vi "PH_Cont-601k_PSU.Set Device Readyness.vi"(0 "VI in":refnum<vi>, 2 "Readyness Device to set":T1, 5 "error in (no error)":errorcluster) -> (14 "VI out":refnum<vi>, 19 "error out":errorcluster)   [LabVIEW 2014, in "PH_Cont-601k_PSU.lvlib"]
doc: "This VI sets the Device readyness to own oattributes and indicates it at the GUI."
uses:
  PH_Cont-601k_PSU.lvlib
  PH_Cont-601k_PSU.Readyness Device.ctl
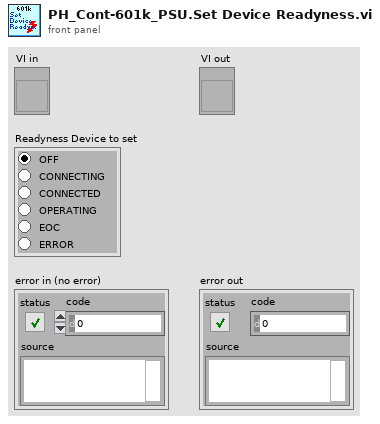
[diagram p1: front panel]
types:
  T1 = typedef "PH_Cont-601k_PSU.lvlib/PH_Cont-601k_PSU.Readyness Device.ctl" = enum32{"OFF", "CONNECTING", "CONNECTED", "OPERATING", "EOC", "ERROR"}
  T2 = typedef "PH_Cont-601k_PSU.lvlib/PH_Cont-601k_PSU.i attribute.ctl" = cluster{"GUI Refs":T3, "Interlock":bool, "Service ID applied Voltage":i32, "Device Settings":cluster{"Configuration":T4, "Flash Interval [s]":dbl, "Mode":T5, "Voltage [V]":u16, "Charge":bool, "VISA resource name":refnum<visa-resource-name>}, "Readyness":T6, "Information":cluster{"VISA resource name":refnum<visa-resource-name>, "Tagname Power On":string, "Interlock":cluster{"Instance":string, "Tagname":string}, "Limits [V]":cluster{"Lower":dbl, "Upper":dbl}, "Tagname PSU On":string}, "R2S":bool, "Charge is allowed":bool}
  T3 = typedef "PH_Cont-601k_PSU.lvlib/PH_Cont-601k_PSU.GUI Refs.ctl" = cluster{"Power On":refnum<vi>, "Hard- and Software":refnum<vi>, "Device Status":refnum<vi>, "Device Error":refnum<vi>, "Configuration":refnum<vi>, "Flash Interval [s]":refnum<vi>, "Interlock":refnum<vi>, "Interlock Indicator":refnum<vi>, "Voltage [V]":refnum<vi>, "Readyness":refnum<vi>, "Mode":refnum<vi>, "Reset Error":refnum<vi>, "Expert working":refnum<vi>, "Charge":refnum<vi>, "PSU On":refnum<vi>}
  T4 = typedef "PH_Cont-601k_PSU.lvlib/PH_Cont-601k_PSU.Configuration.ctl" = u16
  T5 = typedef "PH_Cont-601k_PSU.lvlib/PH_Cont-601k_PSU.Mode.ctl" = enum32{"STOP", "STANDBY", "READY", "EMISSION", "ERROR"}
  T6 = typedef "PH_Cont-601k_PSU.lvlib/PH_Cont-601k_PSU.Readyness.ctl" = cluster{"Program":T7, "Device":T1}
  T7 = typedef "PH_Cont-601k_PSU.lvlib/PH_Cont-601k_PSU.Readyness Program.ctl" = enum32{"OFF", "POWER", "INTERLOCK"}
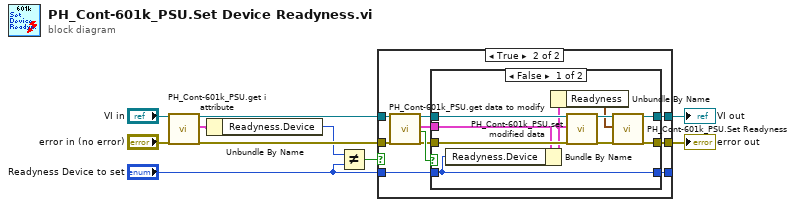
[diagram p0: block diagram]
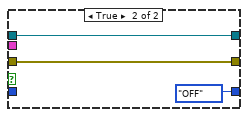
[diagram p3: hidden frame]
diagram:
  n1 = call "PH_Cont-601k_PSU.get i attribute.vi"("i ref in"="VI in", "error in (no error)"="error in (no error)") -> ("i ref out"=w5:refnum<vi>, "i attribute"=w4:T2, "error out"=w7:errorcluster)  [unwired: 15 in]
  n2 = Unbundle By Name(w4) -> ("Readyness.Device"=w3:T1)
  n3 = Not Equal?(x=w3, y="Readyness Device to set") -> (x != y?=w1:bool)
  n4 = case shown="True" w1 {
    tunnel: [w13 w21] -> w10
    tunnel: [w12 w19] -> w9
    tunnel: [w11 w17] -> _
    tunnel: w7 -> [w12 w16]
    tunnel: w5 -> [w13 w15]
    tunnel: "Readyness Device to set" -> [w11 w14]
    frame False {
    }
    frame True {
      n5 = call "PH_Cont-601k_PSU.get data to modify.vi"("i ref in"=w15, "error in (no error)"=w16) -> ("i ref out"=w20:refnum<vi>, "i attribute"=w23:T2, "timed out"=w22:bool, "error out"=w18:errorcluster)  [unwired: 14 in]
      n6 = case shown="False" w22 {
        tunnel: w18 -> [w33 w35]
        tunnel: [w31 w35] -> w19
        tunnel: w20 -> [w30 w36]
        tunnel: [w28 w36] -> w21
        tunnel: w23 -> [w27 _]
        tunnel: w14 -> [w24 _]
        tunnel: [w24 PH_Cont-601k_PSU.Readyness_Device."OFF" ("Readyness Device")] -> w17
        frame False {
          n7 = Bundle By Name(cluster=w27, "Readyness.Device"=w24) -> (w26:T2)
          n8 = Unbundle By Name(w26) -> ("Readyness"=w25:T6)
          n9 = call "PH_Cont-601k_PSU.set modified data.vi"("i ref in"=w30, "i attribute"=w26, "error in (no error)"=w33) -> ("i ref out"=w29:refnum<vi>, "error out"=w32:errorcluster)  [unwired: 15 in]
          n10 = call "PH_Cont-601k_PSU.Set Readyness.vi"("VI in"=w29, "Current Readyness"=w25, "error in (no error)"=w32) -> ("VI out"=w28:refnum<vi>, "error out"=w31:errorcluster)  [unwired: 15 in]
        }
        frame True {
        }
      }
    }
  }
  "VI out" <- w10
  "error out" <- w9
